vi "Write Part ID.vi"(8 "error in (no error)":errorcluster, 10 "Part ID":string, 11 "Thermistor in":refnum<class "Thermistor.lvclass">) -> (0 "error out":errorcluster, 3 "Thermistor out":refnum<class "Thermistor.lvclass">)   [LabVIEW 2024, in "Thermistor.lvclass"]
uses:
  Thermistor.lvclass
  Thermistor.lvclass/Thermistor.ctl
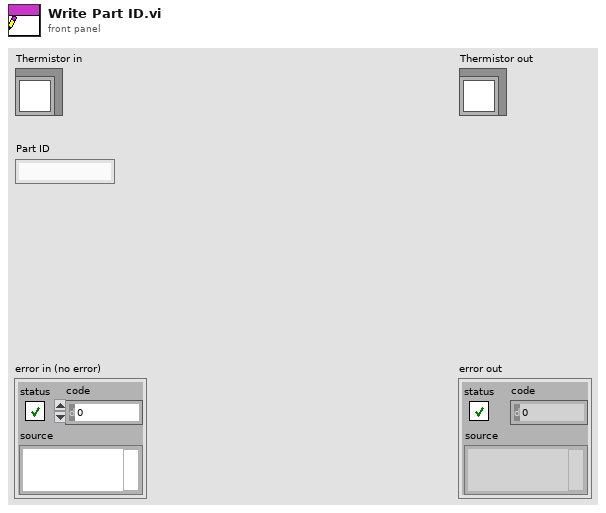
[diagram p1: front panel]
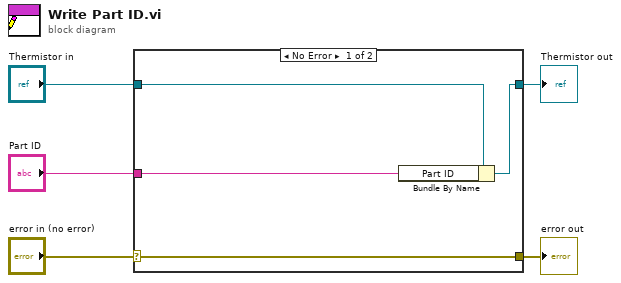
[diagram p0: block diagram]
diagram:
  n1 = case shown="No Error" "error in (no error)" {
    selector: "error in (no error)" -> [w9 w10]
    tunnel: [w9 w10] -> w4
    tunnel: [w7 w11] -> w2
    tunnel: "Thermistor in" -> [w8 w11]
    tunnel: "Part ID" -> [w6 _]
    frame No Error {
      n2 = Bundle By Name(cluster=w8, "Part ID"=w6) -> (w7:refnum<class "Thermistor.lvclass">)
    }
    frame Error {
    }
  }
  "error out" <- w4
  "Thermistor out" <- w2
